vi "CylGet.vi"(8 "error in (no error)":errorcluster, 11 "Cycle in":refnum<class "Cycle.lvclass">) -> (0 "error out":errorcluster, 1 "Tag":string, 2 "SEQ Pool":T1(array[cluster]), 3 "Cycle out":refnum<class "Cycle.lvclass">, 4 "Cycle on":dbl[unit], 6 "Cycle off":dbl[unit])   [LabVIEW 2012, in "Cycle.lvclass"]
uses:
  Cycle.lvclass
  Sequence.lvclass
  Cycle.lvclass/Cycle.ctl
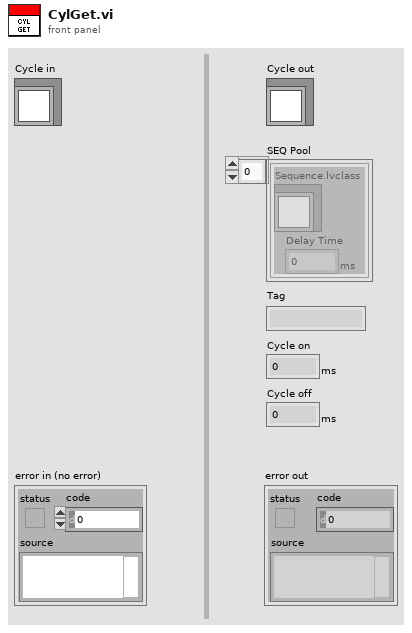
[diagram p1: front panel]
types:
  T1 = cluster{"Sequence.lvclass":refnum<class "Sequence.lvclass">, "Delay Time":dbl[unit]}[]
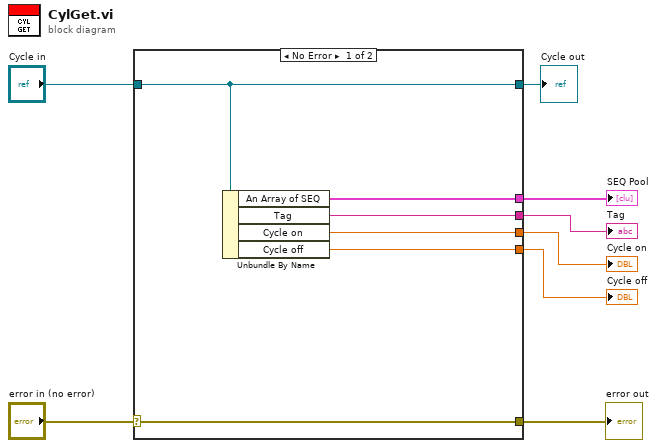
[diagram p0: block diagram]
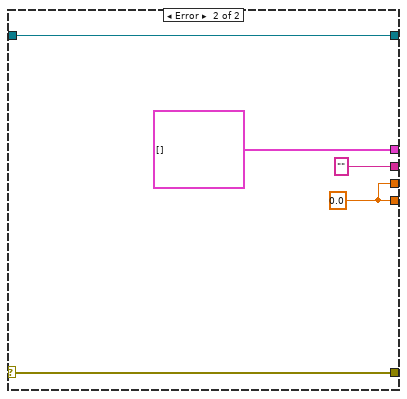
[diagram p2: hidden frame]
diagram:
  n1 = case shown="No Error" "error in (no error)" {
    selector: "error in (no error)" -> [w14 w18]
    tunnel: [w14 w18] -> w7
    tunnel: [w13 w19] -> w5
    tunnel: "Cycle in" -> [w13 w19]
    tunnel: [w12 "" ("Tag")] -> w4
    tunnel: [w11 w16] -> w2
    tunnel: [w10 w16] -> w3
    tunnel: [w9 T1 [] ("An Array of SEQ")] -> w1
    frame No Error {
      n2 = Unbundle By Name(w13) -> ("An Array of SEQ"=w9:T1, "Tag"=w12:string, "Cycle on"=w11:dbl[unit], "Cycle off"=w10:dbl[unit])
    }
    frame Error {
      w16 = dbl[unit] 0.0 ("Cycle on")
    }
  }
  "error out" <- w7
  "Cycle out" <- w5
  "Tag" <- w4
  "Cycle off" <- w3
  "Cycle on" <- w2
  "SEQ Pool" <- w1
